vi "Construct City.vi"(5 "City In":refnum<class "City.lvclass">, 8 "error in (no error)":errorcluster, 9 "Weather Forecast":refnum<class "Weather Forecast.lvclass">, 10 "Population":u32, 11 "Name":string) -> (0 "error out":errorcluster, 3 "City":refnum<class "City.lvclass">)   [LabVIEW 2017, in "Generic Object Serializer Tests.lvlib" / "City.lvclass"]
uses:
  City.lvclass
  Weather Forecast/Weather Forecast.lvclass
  City.lvclass/City.ctl
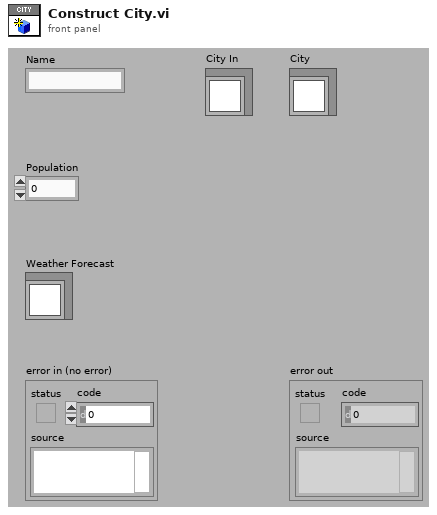
[diagram p1: front panel]
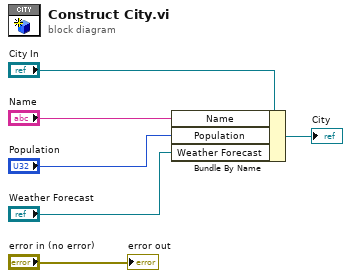
[diagram p0: block diagram]
diagram:
  n1 = Bundle By Name(cluster="City In", "Name"="Name", "Population"="Population", "Weather Forecast"="Weather Forecast") -> (→"City":refnum<class "City.lvclass">)
  "error out" <- "error in (no error)"
